vi "from string.vi"(8 "error in":errorcluster, 9 "data":string, 10 "version":string, 11 "sample module configuration in":refnum<class "sample module configuration.lvclass">) -> (0 "error out":errorcluster, 3 "sample module configuration out":refnum<class "sample module configuration.lvclass">)   [LabVIEW 2013, in "sample module configuration.lvclass"]
doc: "Provides an interface for loading a module configuration from a file or other serialized data source. It is recommended that all children of this class store data in two sets--data required for its own initialization, and any data required for parent initialization--and that each implementation uses the <b>Call Parent Method</b> primitive to de-serialize parent information. As a result, it is expected that every module configuration class calls <b>component configuration.lvclass:From String.vi</b>."
uses:
  sample module configuration.lvclass
  channel/TBM channel.lvclass
  sample module configuration.lvclass/sample module configuration.ctl
  module configuration/TBM module configuration.lvclass
  root configuration/TBM configuration.lvclass
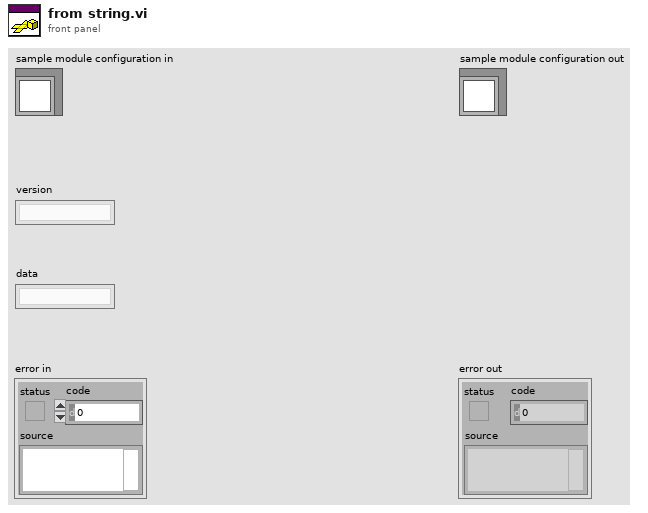
[diagram p1: front panel]
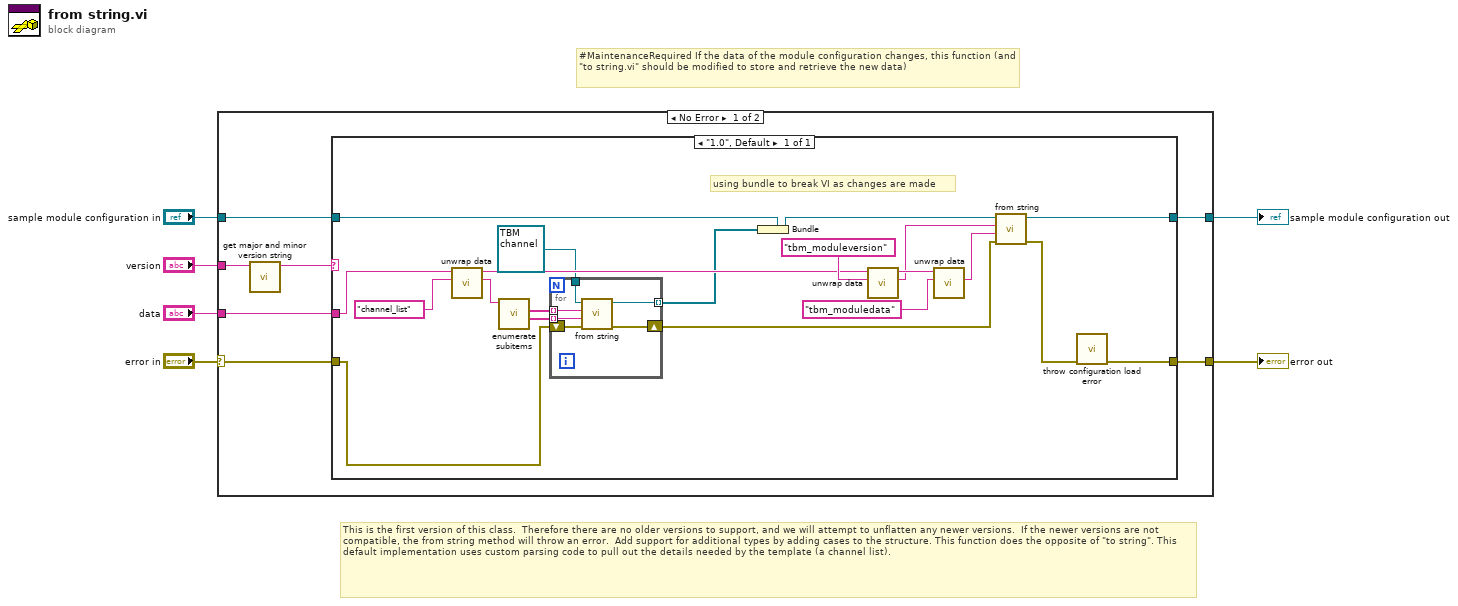
[diagram p0: block diagram]
diagram:
  # "#MaintenanceRequired If the data of the module configuration changes, this function (and \"to string.vi\" should be modified to store and retrieve the new data)"
  # "This is the first version of this class.  Therefore there are no older versions to support, and we will attempt to unflatten any newer versions.  If the newer versions are not compatible, the from string method will throw an error.  Add support for additional types by adding cases to the structure. This function does the opposite of \"to string\". This default implementation uses custom parsing code to pull out the details needed by the template (a channel list)."
  n1 = case shown="No Error" "error in" {
    selector: "error in" -> [w7 w41]
    tunnel: "data" -> [w13 _]
    tunnel: "sample module configuration in" -> [w12 w40]
    tunnel: [w11 w40] -> w5
    tunnel: [w10 w41] -> w4
    tunnel: "version" -> [w9 _]
    frame No Error {
      n2 = call "get major and minor version string.vi"("full version"=w9) -> ("major.minor version"=w8:string)  [unwired: 10 in]
      n3 = case shown="\"1.0\", Default" w8 {
        tunnel: w13 -> [w22]
        tunnel: w7 -> [w17]
        tunnel: w12 -> [w33]
        tunnel: [w32] -> w11
        tunnel: [w30] -> w10
        frame "1.0", Default {
          # "using bundle to break VI as changes are made"
          n4 = call "unwrap data.vi"("identifier"="channel_list" ("additional identifier"), "data to unwrap"=w22) -> ("unwrapped data"=w20:string, "remaining string"=w25:string)  [unwired: 8 in]
          n5 = call "enumerate subitems.vi"("data to enumerate"=w20) -> ("associated data"=w18:string[], "discovered subitems"=w19:string[])  [unwired: 8 in, 1 out]
          n6 = for {
            tunnel: w19 -> [w39] mode=indexing
            tunnel: w18 -> [w38] mode=indexing
            shift-right: [w37] -> w16
            shift-left: w17 -> [w36]
            tunnel: [w35] -> w15 mode=indexing
            tunnel: refnum<class "TBM channel.lvclass"> refnum ("channel in") -> [w34]
            n7 = call-dynamic "from string.vi"("error in"=w36, "channel data"=w38, "identifier"=w39, "channel in"=w34) -> ("error out"=w37:errorcluster, "channel out"=w35:refnum<class "TBM channel.lvclass">)  [unwired: 6 in]
          }
          n8 = Bundle(cluster=w33, w15) -> (w21:refnum<class "sample module configuration.lvclass">)
          n9 = call "unwrap data.vi"("identifier"="tbm_moduleversion" ("additional identifier"), "data to unwrap"=w25) -> ("unwrapped data"=w24:string, "remaining string"=w27:string)  [unwired: 8 in]
          n10 = call "unwrap data.vi"("identifier"="tbm_moduledata" ("additional identifier"), "data to unwrap"=w27) -> ("unwrapped data"=w23:string)  [unwired: 8 in, 1 out]
          n11 = call-parent "from string.vi"("error in"=w16, "data"=w23, "version"=w24, "module configuration in"=w21) -> ("error out"=w31:errorcluster, "module configuration out"=w32:refnum<class "sample module configuration.lvclass">)  [unwired: 6 in]
          n12 = call "throw configuration load error.vi"("error in"=w31) -> ("error out"=w30:errorcluster)  [unwired: 10 in]
        }
      }
    }
    frame Error {
    }
  }
  "error out" <- w4
  "sample module configuration out" <- w5
